vi "Control - PID Control.vi"() -> ()   [LabVIEW 2013, in "PID Control Workspace Object.lvlib"]
doc: "Sample numeric display item."
uses:
  Control Workspace Object Support.llb/PID Control Workspace Object.lvlib
  NationalInstruments.VeriStand.SystemStorage
  NationalInstruments.VeriStand.ClientAPI
  Control Workspace Object Support.llb/Constants.vi
  Control Workspace Object Support.llb/Control Addon Shared.lvlib
  Control Workspace Object Support.llb/NI_VS Workspace ExecutionAPI.lvlib
panel:
  in  "Manual Output":dbl
  in  "Manual Control":bool
  in  "Setpoint":dbl
  in  "NIVS.System Definition Root":refnum<k24>
  in  "NIVS.Gateway IP Address":string
  in  "Hold":bool
  in  "Autoscale Y":bool=TRUE
  in  "Autoscale X":bool=TRUE
  out "Chart":waveform(dbl)[](graph)
  out "Control Name":string
  in  "Item.Data":T1
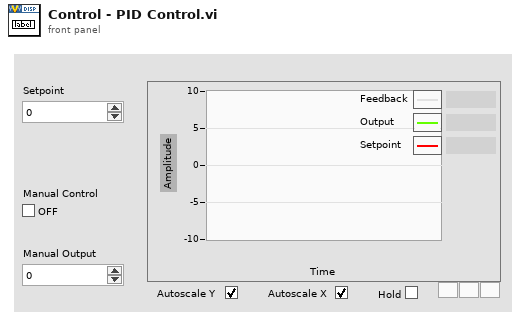
[diagram p1: front panel]
types:
  T1 = cluster{"Template VI":string, "Position X":i32, "Position Y":i32, "Custom":string, "Show Title Bar":bool, "ID":i32, "Always On Top":bool, "Allow Resize":bool, "Allow Minimize":bool, "Allow Close":bool, "Size to Screen":bool, "Screen.ID":i32, "State":enum16{"Normal", "New"}, "Title":string, "Window Bounds":cluster{"[0]":i16, "[1]":i16, "[2]":i16, "[3]":i16}, "Channel Ref":u64, "Unit":string, "Default Units?":bool, "Flash Limit?":bool, "Color 1":u32, "Color 2":u32, "Color 3":u32, "Color 4":u32, "Bck Color":u32, "Fore Color":u32, "Limit 1":dbl, "Limit 2":dbl, "Limit 3":dbl, "Limit 4":dbl, "Limit Mode 1":i32, "Limit Mode 2":i32, "Limit Mode 3":i32, "Limit Mode 4":i32, "Scale Precision":i32, "Scale Min":dbl, "Scale Max":dbl, "Format":i32, "Precision":i32, "Background Type":i32, "IDs":i32[], "Units":string[], "Labels":string[], "Scale Factor":dbl, "Scale Offset":dbl, "YScale Index":u32[], "XScale":cluster{"Format":u8, "Precision":u8, "Fit":u8, "Label":string, "Use Default Label":bool, "Label Visible":bool, "Min":dbl, "Max":dbl}, "YScales":cluster{"Format":u8, "Precision":u8, "Fit":u8, "Label":string, "Use Default Label":bool, "Label Visible":bool, "Min":dbl, "Max":dbl}[], "Plots":cluster{"Bar Style":u8, "Fill To":i16, "Fill/PtColor":u32, "Line Style":u8, "Line Width":u8, "Color":u32, "Interp":u8, "Point Style":u8}[], "Update Period":dbl, "History Length":dbl, "My.Ref":refnum<vi>, "Is Control?":bool, "Channel Paths":string[], "Custom Data":variant}
  T2 = enum8{"Idle", "Start Acq", "Run", "Stop Acq", "Exit"}
  T3 = cluster{"Action":enum8{"Idle", "Start Acq", "Run", "Stop Acq", "Exit"}, "Channels":string[]}
  T4 = cluster{"Initialized Waveform":waveform(dbl)[], "VS UDP Session":refnum<k24>, "Channel IDs":i32[], "Packet IDs":i32[], "Max Packet Size":i32, "UDP Ref":refnum<k16>}
  T5 = cluster{"Cached":cluster{"Path":string}, "Found?":bool, "UDP Channels":string[], "Connected?":bool, "Previous Values":dbl[], "Slow Channels":string[]}
  T6 = cluster{"Operation":enum16{"SetCustomData", "DeleteItem"}, "Data":variant}
  T7 = cluster{"CustDatRef":refnum<user-event>, "EvtRef":refnum<k27>}
  T8 = cluster{"Event Registration Refnum":refnum<event-registration>, "SystemChangeEventRef":refnum<event-registration>}
  T9 = cluster{"ID":i32, "t0":dbl, "dt":dbl, "Channel IDs":i32[], "Channel Data":dbl[][], "Sample Offset":u64}
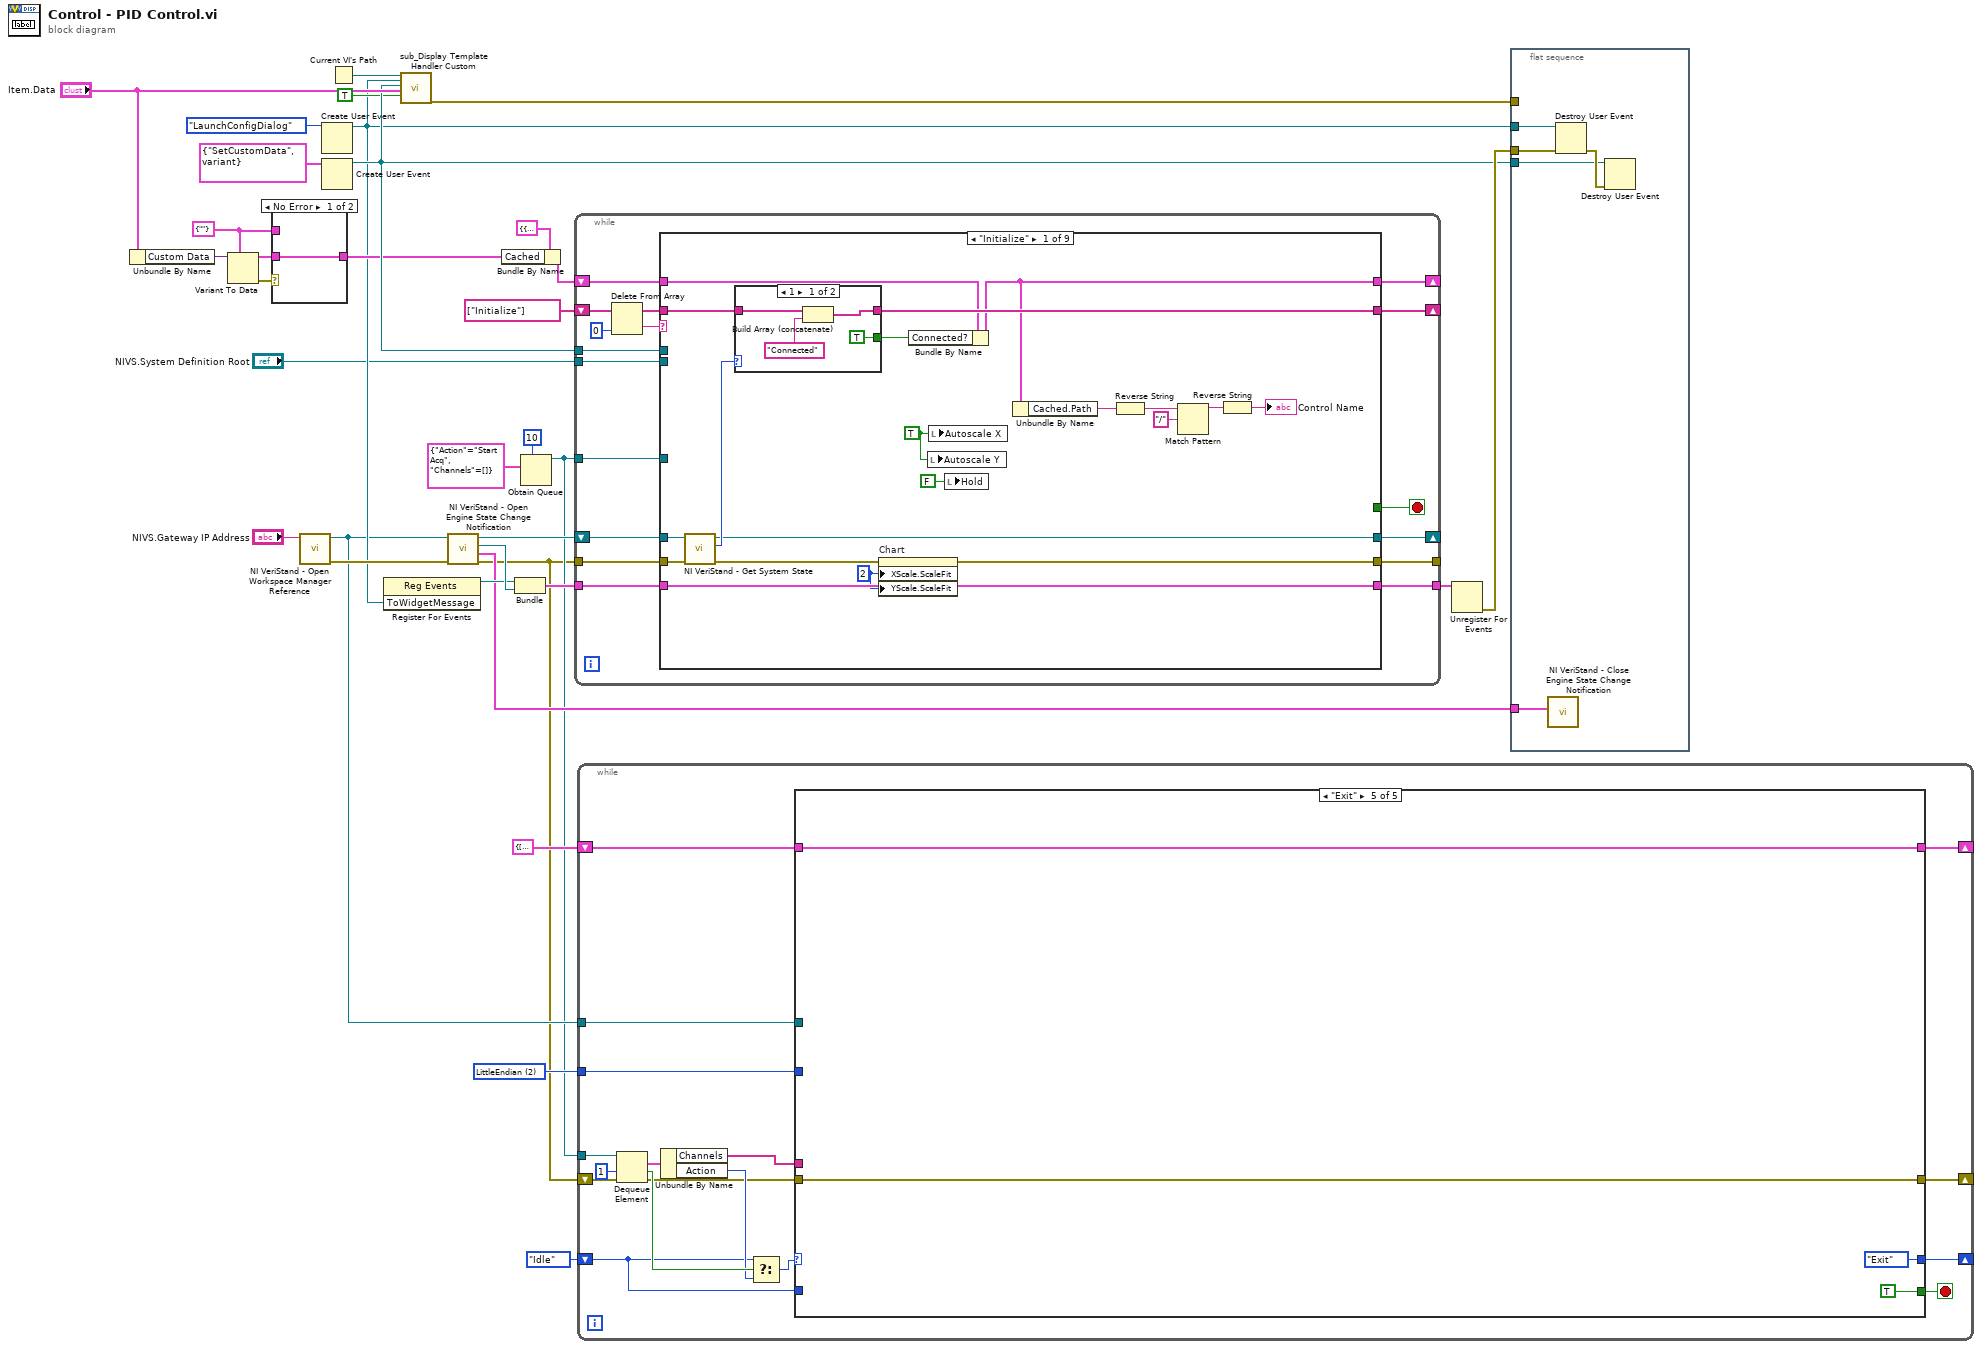
[diagram p0: block diagram]
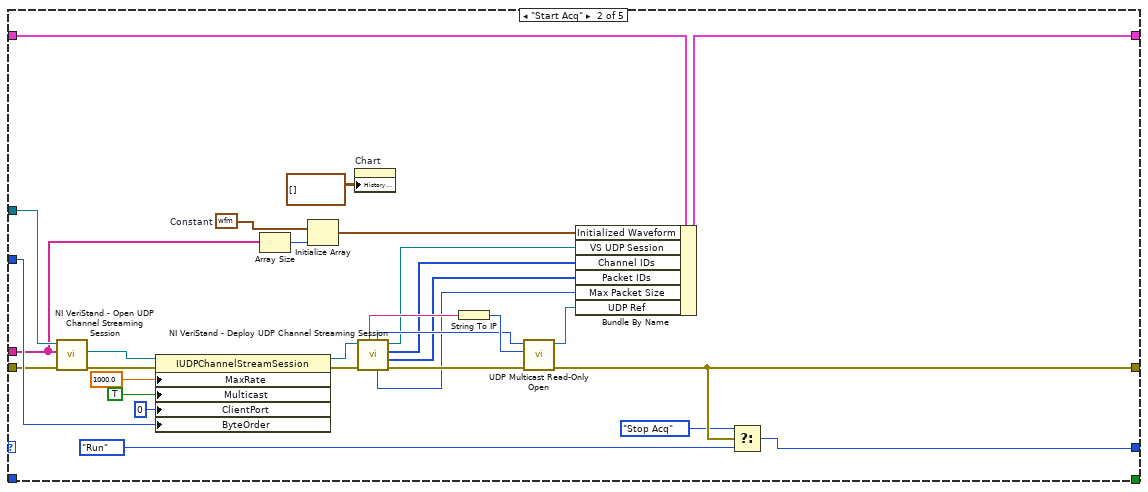
[diagram p3: hidden frame]
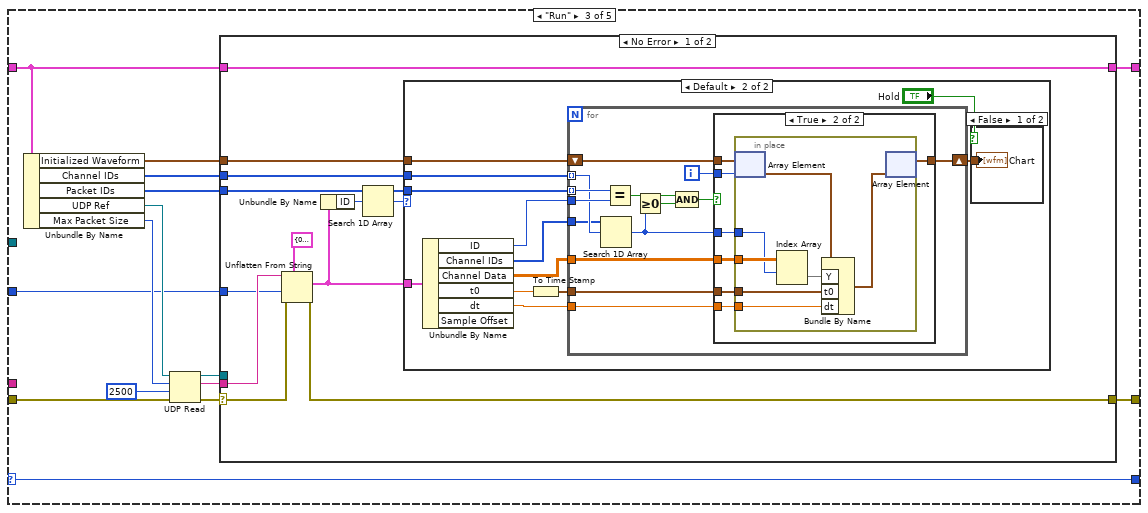
[diagram p4: hidden frame]
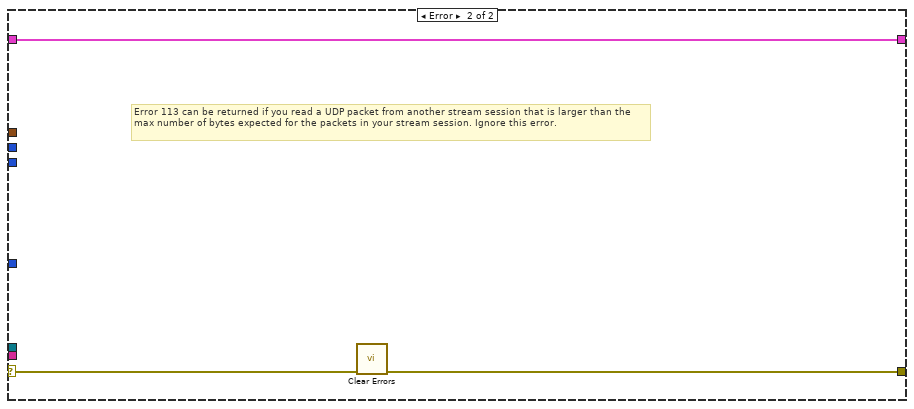
[diagram p8: hidden frame]
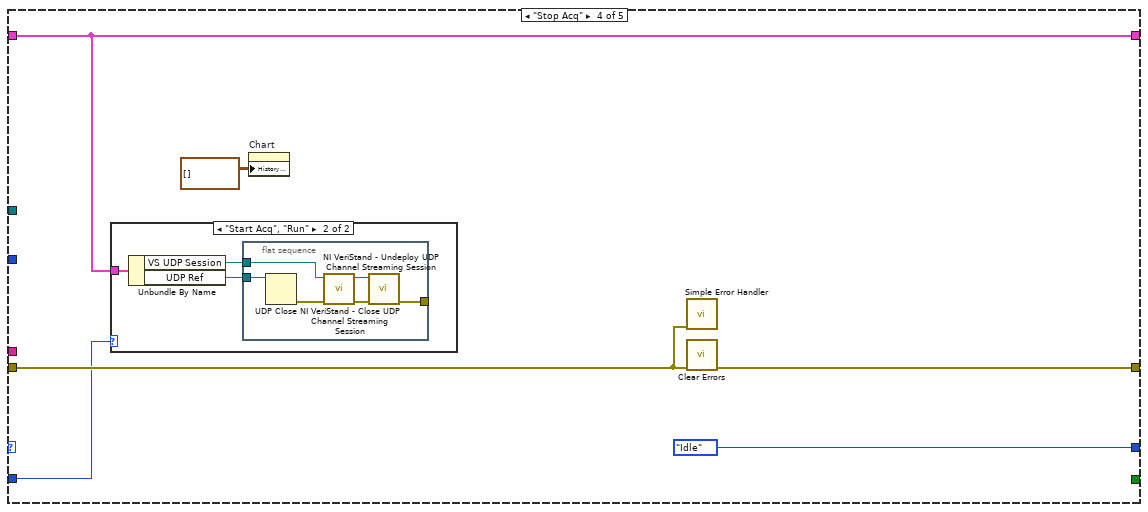
[diagram p9: hidden frame]
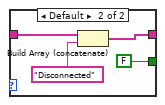
[diagram p12: hidden frame]
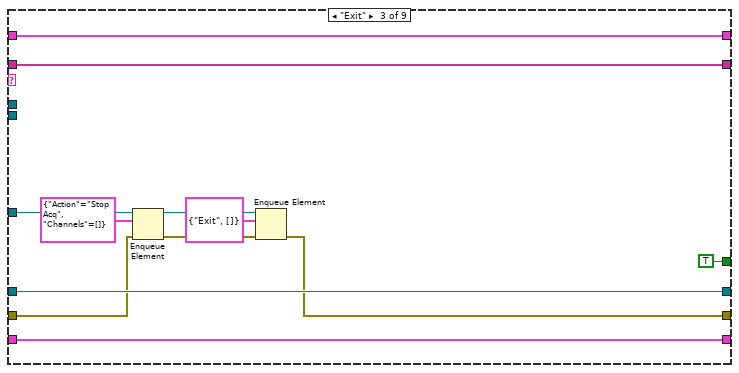
[diagram p14: hidden frame]
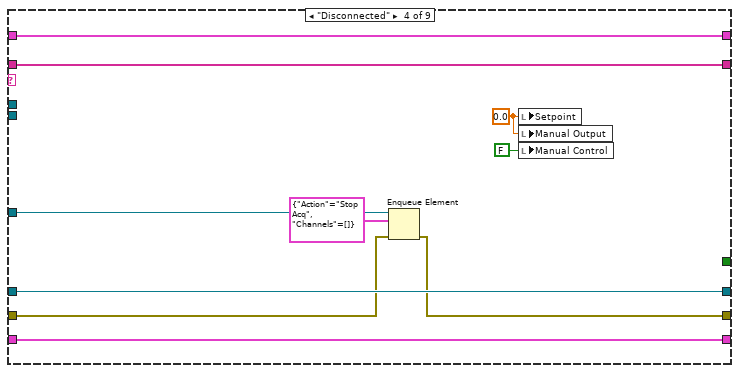
[diagram p15: hidden frame]
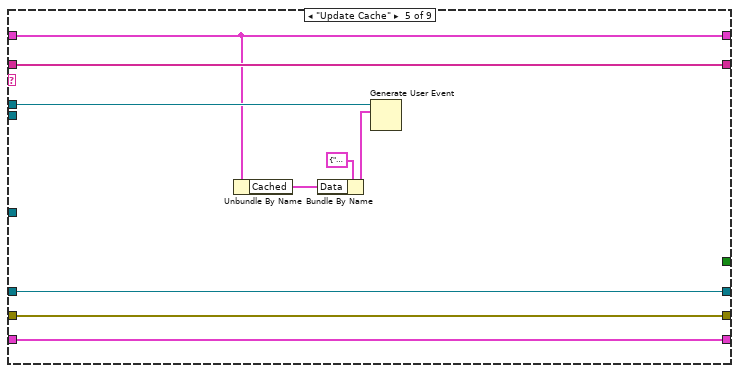
[diagram p16: hidden frame]
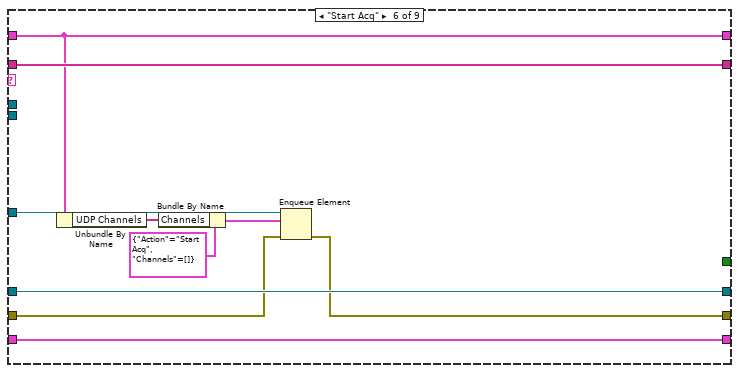
[diagram p17: hidden frame]
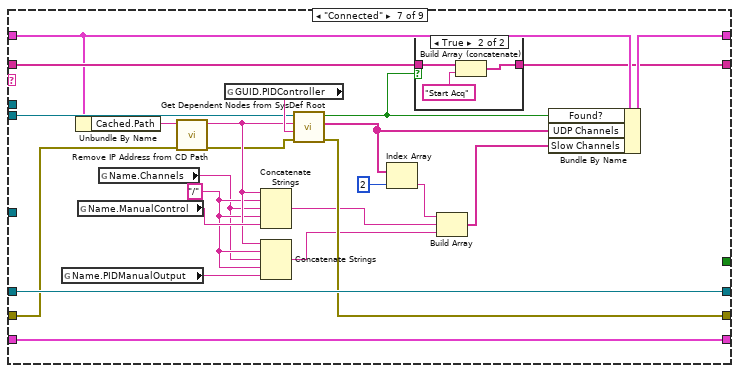
[diagram p18: hidden frame]
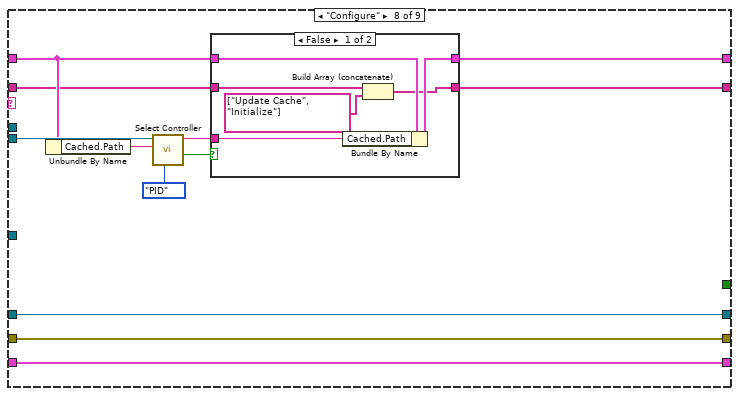
[diagram p20: hidden frame]
diagram:
  w6 = 2 items=["BigEndian", "NativeHostOrder", "LittleEndian"] ("Byte Order")
  w14 = cluster{"Path":string} {"Path"=""}
  n1 = Unbundle By Name("Item.Data") -> ("Custom Data"=w18:variant)
  n2 = Variant To Data(type=w14, Variant=w18) -> (data=w15:cluster{"Path":string}, error out=w16:errorcluster)  [unwired: 1 in]
  n3 = case shown="No Error" w16 {
    tunnel: w15 -> [w35 _]
    tunnel: [w35 w36] -> w11
    tunnel: w14 -> [_ w36]
    frame No Error {
    }
    frame Error {
    }
  }
  n4 = call "NI VeriStand - Open Workspace Manager Reference.vi"("Gateway IP Address (\"\": localhost)"="NIVS.Gateway IP Address") -> ("error out"=w25:errorcluster, "WorkspaceManager"=w8:refnum<k24>)  [unwired: 9 in]
  n5 = Create User Event(user event datatype=enum16{"Stop", "LaunchConfigDialog"}."LaunchConfigDialog" ("ToWidgetMessage")) -> (user event=w10:refnum<user-event>)  [unwired: 1 in, 1 out]
  n6 = Create User Event(user event datatype=T6 {"Operation"=enum."SetCustomData", "Data"=variant} ("Data")) -> (user event=w28:refnum<user-event>)  [unwired: 1 in, 1 out]
  n7 = Current VI's Path() -> (path=w30:path)
  n8 = register-events(w10) -> (reference out=w23:refnum<event-registration>)  [unwired: 2 in, 1 out]
  n9 = call "sub_Display Template Handler Custom.vi"("Parent.Path"=w30, "ToWidgetEvent"=w10, "ToWorkspace"=w28, "Item.Data"="Item.Data", "Resizable"=TRUE) -> ("error out"=w34:errorcluster)  [unwired: 14 in]
  n10 = call "NI VeriStand - Open Engine State Change Notification.vi"("error in (no error)"=w25, "WorkspaceManager in"=w8) -> ("error out"=w1:errorcluster, "SystemStateRefs"=w21:T7, "SystemChangeEventRef"=w24:refnum<event-registration>, "WorkspaceManager out"=w19:refnum<k24>)  [unwired: 6 in]
  n11 = Bundle By Name(cluster=T5 {"Cached"={"Path"=""}, "Found?"=FALSE, "UDP Channels"=[], "Connected?"=FALSE, "Previous Values"=[0.0, 0.0, 0.0], "Slow Channels"=[]}, "Cached"=w11) -> (w12:T5)
  n12 = Bundle("Event Registration Refnum"=w23, "SystemChangeEventRef"=w24) -> (w22:T8)  [unwired: 1 in]
  n13 = Obtain Queue(max queue size (-1, unlimited)=10, element data type=T3 {"Action"=enum."Start Acq", "Channels"=[]}) -> (queue out=w3:refnum<queue>)  [unwired: 3 in, 2 out]
  n14 = while {
    tunnel: w22 -> [w53]
    tunnel: w28 -> [w51]
    shift-right: [w45] -> _
    shift-left: string[] ["Initialize"] -> [w49]
    shift-right: [w43] -> _
    shift-left: w19 -> [w42]
    tunnel: w1 -> [w47]
    tunnel: [w44] -> w17
    tunnel: [w40] -> _
    shift-right: [w39] -> _
    shift-left: w12 -> [w41]
    tunnel: "NIVS.System Definition Root" -> [w38]
    tunnel: w3 -> [w37]
    stop <- w52 stop-if-true
    n15 = Delete From Array(array=w49, index=0) -> (deleted portion=w48:string, array with subset deleted=w46:string[])  [unwired: 1 in]
    n16 = case shown="\"Initialize\"" w48 {
      tunnel: w53 -> [w67 w85 w97 w107 w116 w126 w150 w167 w186]
      tunnel: [_ _ TRUE _ _ _ _ _ _] -> w52
      tunnel: [w69 w86 w98 w108 w117 w127 w133 w157 w183] -> w45
      tunnel: w51 -> [_ _ _ _ w113 _ _ _ _]
      tunnel: w47 -> [w72 w83 w89 w103 w114 w119 w137 w165 w179]
      tunnel: w46 -> [w70 w86 w98 w108 w117 w127 w151 w156 w182]
      tunnel: [w67 w85 w97 w107 w116 w126 w150 w167 w184] -> w44
      tunnel: [w68 w84 w96 w106 w115 w125 w149 w166 w180] -> w43
      tunnel: w42 -> [w71 w84 w96 w106 w115 w125 w149 w166 w181]
      tunnel: w41 -> [w61 w82 w95 w105 w110 w124 w145 w161 w176]
      tunnel: [w55 w83 w88 w102 w114 w118 w148 w165 w178] -> w40
      tunnel: [w60 w82 w95 w105 w110 w124 w144 w160 w177] -> w39
      tunnel: w38 -> [_ _ _ _ _ _ w146 w163 _]
      tunnel: w37 -> [_ _ w94 w104 _ w123 _ _ _]
      frame "Initialize" {
        w57 = u8 2 ("X Scale.Scale Fit")
        w58 = TRUE ("Autoscale X")
        n17 = call "NI VeriStand - Get System State.vi"("error in (no error)"=w72, "WorkspaceManager in"=w71) -> ("error out"=w56:errorcluster, "System State"=w73:u8, "WorkspaceManager  out"=w68:refnum<k24>)  [unwired: 5 in, 2 out]
        n18 = case shown="1" w73 {
          tunnel: w70 -> [w77 w81]
          tunnel: [w76 w80] -> w69
          tunnel: [TRUE FALSE] -> w59
          frame 1 {
            n19 = Build Array (concatenate)(w77, "Connected") -> (w76:string[])
          }
          frame Default {
            n20 = Build Array (concatenate)(w81, "Disconnected") -> (w80:string[])
          }
        }
        n21 = property on="Chart" class="WFChart (strict)"(error in=w56, "XScale.ScaleFit"=w57, "YScale.ScaleFit"=w57) -> (error out=w55:errorcluster)  [unwired: 1 in, 1 out]
        n22 = Bundle By Name(cluster=w61, "Connected?"=w59) -> (w60:T5)
        n23 = local write "Autoscale Y"(w58) -> ()
        n24 = local write "Autoscale X"(w58) -> ()
        n25 = local write "Hold"(FALSE ("Hold")) -> ()
        n26 = Unbundle By Name(w60) -> ("Cached.Path"=w63:string)
        n27 = Reverse String(1:w63) -> (0:w66:string)
        n28 = Match Pattern(string=w66, regular expression="/") -> (before substring=w62:string)  [unwired: 1 in, 3 out]
        n29 = Reverse String(1:w62) -> (0:→"Control Name":string)
      }
      frame Default {
      }
      frame "Exit" {
        n30 = Enqueue Element(queue=w94, element=T3 {"Action"=enum."Stop Acq", "Channels"=[]}, error in (no error)=w89) -> (queue out=w92:refnum<queue>, error out=w90:errorcluster)  [unwired: 1 in, 1 out]
        n31 = Enqueue Element(queue=w92, element=T3 {"Action"=enum."Exit", "Channels"=[]}, error in (no error)=w90) -> (error out=w88:errorcluster)  [unwired: 1 in, 2 out]
      }
      frame "Disconnected" {
        w100 = 0.0 ("Setpoint")
        n32 = Enqueue Element(queue=w104, element=T3 {"Action"=enum."Stop Acq", "Channels"=[]}, error in (no error)=w103) -> (error out=w102:errorcluster)  [unwired: 1 in, 2 out]
        n33 = local write "Setpoint"(w100) -> ()
        n34 = local write "Manual Output"(w100) -> ()
        n35 = local write "Manual Control"(FALSE ("Manual Control")) -> ()
      }
      frame "Update Cache" {
        n36 = Unbundle By Name(w110) -> ("Cached"=w109:cluster{"Path":string})
        n37 = Bundle By Name(cluster=T6 {"Operation"=enum."SetCustomData", "Data"=variant} ("event data"), "Data"=w109) -> (w111:T6)
        n38 = Generate User Event(user event=w113, event data cluster=w111) -> ()  [unwired: 2 in, 2 out]
      }
      frame "Start Acq" {
        n39 = Unbundle By Name(w124) -> ("UDP Channels"=w121:string[])
        n40 = Bundle By Name(cluster=T3 {"Action"=enum."Start Acq", "Channels"=[]}, "Channels"=w121) -> (w120:T3)
        n41 = Enqueue Element(queue=w123, element=w120, error in (no error)=w119) -> (error out=w118:errorcluster)  [unwired: 1 in, 2 out]
      }
      frame "Connected" {
        w130 = "/" ("string")
        n42 = global read "Constants.vi" "Name.PIDManualOutput"() -> (w140:string)
        n43 = Unbundle By Name(w145) -> ("Cached.Path"=w143:string)
        n44 = global read "Constants.vi" "Name.ManualControl"() -> (w142:string)
        n45 = global read "Constants.vi" "Name.Channels"() -> (w129:string)
        n46 = call "Remove IP Address from CD Path.vi"("error in (no error)"=w137, "CD Path"=w143) -> ("error out"=w136:errorcluster, "Path"=w141:string)  [unwired: 8 in]
        n47 = global read "Constants.vi" "GUID.PIDController"() -> (w147:string)
        n48 = Concatenate Strings(w141, w130, w129, w130, w142) -> (w139:string)
        n49 = Concatenate Strings(w141, w130, w129, w130, w140) -> (w138:string)
        n50 = call "Get Dependent Nodes from SysDef Root.vi"("error in (no error)"=w136, "GUID"=w147, "Path"=w141, "SysDef Ref"=w146) -> ("error out"=w148:errorcluster, "Channels"=w132:string[], "Found"=w128:bool)  [unwired: 5 in]
        n51 = Index Array(array=w132, index=2) -> (element=w134:string)
        n52 = case shown="True" w128 {
          tunnel: w151 -> [w152 w155]
          tunnel: [w152 w154] -> w133
          frame False {
          }
          frame True {
            n53 = Build Array (concatenate)(w155, "Start Acq") -> (w154:string[])
          }
        }
        n54 = Build Array(w134, w139, w138) -> (w131:string[])
        n55 = Bundle By Name(cluster=w145, "Found?"=w128, "UDP Channels"=w132, "Slow Channels"=w131) -> (w144:T5)
      }
      frame "Configure" {
        n56 = Unbundle By Name(w161) -> ("Cached.Path"=w162:string)
        n57 = call "Select Controller.vi"("Type"=enum16{"PID", "Industrial"}."PID", "CD Path"=w162, "NIVS.System Definition Root"=w163) -> ("Cancelled?"=w159:bool, "Custom Device Path Out"=w158:string)  [unwired: 6 in, 1 out]
        n58 = case shown="False" w159 {
          tunnel: w161 -> [w173 w174]
          tunnel: [w172 w174] -> w160
          tunnel: w158 -> [w171 _]
          tunnel: [w169 w175] -> w157
          tunnel: w156 -> [w170 w175]
          frame False {
            n59 = Bundle By Name(cluster=w173, "Cached.Path"=w171) -> (w172:T5)
            n60 = Build Array (concatenate)(w170, string[] ["Update Cache", "Initialize"]) -> (w169:string[])
          }
          frame True {
          }
        }
      }
      frame "" {
        n61 = event shown="[1] \"Autoscale Y\", \"Autoscale X\": Value Change" {
          selector: w186 -> [_ _ _ _ _]
          dyn-events: [_ _ _ _ _] -> w184
          timeout: 100 -> [_ _ _ _ _]
          tunnel: [w203 w225 w242 w271 w291] -> w183
          tunnel: w182 -> [w203 w225 w242 w272 w290]
          tunnel: w181 -> [w200 w224 w235 w275 w292]
          tunnel: [w199 w224 w234 w274 w292] -> w180
          tunnel: w179 -> [w202 w218 w237 w277 w289]
          tunnel: [w201 w217 w236 w276 w289] -> w178
          tunnel: [w196 w223 w230 w269 w288] -> w177
          tunnel: w176 -> [w197 w223 w230 w270 w288]
          event Timeout {
            n62 = event-data() -> ()  [unwired: 2 out]
            n63 = Unbundle By Name(w197) -> ("Found?"=w189:bool, "Connected?"=w195:bool, "Slow Channels"=w198:string[])
            n64 = Compound Arithmetic op=AND(w189, w195) -> (w190:bool)
            n65 = case shown="True" w190 {
              tunnel: w202 -> [w206 w212]
              tunnel: [w206 w211] -> w201
              tunnel: w200 -> [w205 w210]
              tunnel: [w205 w209] -> w199
              tunnel: w198 -> [_ w208]
              tunnel: [dbl[] [0.0, 0.0, 0.0] ("Values") w207] -> w194
              frame False {
              }
              frame True {
                n66 = call "NI VeriStand - Get Multiple Channel Values.vi"("error in (no error)"=w212, "Channels"=w208, "WorkspaceManager in"=w210) -> ("error out"=w211:errorcluster, "Values"=w207:dbl[], "WorkspaceManager out"=w209:refnum<k24>)  [unwired: 6 in]
              }
            }
            n67 = Index Array(array=w194) -> (element #1=w193:dbl, element #2=w188:dbl, element #3=w187:dbl)  [unwired: 3 in]
            n68 = To Long Integer(number=w188) -> (32bit integer=w192:i32)
            n69 = Not Equal To 0?(x=w192) -> (x != 0?=w191:bool)
            n70 = local write "Setpoint"(w193) -> ()
            n71 = local write "Manual Control"(w191) -> ()
            n72 = local write "Manual Output"(w187) -> ()
            n73 = Bundle By Name(cluster=w197, "Previous Values"=w194) -> (w196:T5)
          }
          event "Autoscale Y", "Autoscale X": Value Change {
            n74 = event-data() -> ()  [unwired: 2 out]
            n75 = Select(t=u8 2, s="Autoscale X", f=u8 0 ("X Scale.Scale Fit")) -> (s? t:f=w220:u8)
            n76 = Select(t=u8 2, s="Autoscale Y", f=u8 0 ("X Scale.Scale Fit")) -> (s? t:f=w213:u8)
            n77 = property on="Chart" class="WFChart (strict)"(error in=w218, "XScale.ScaleFit"=w220, "YScale.ScaleFit"=w213) -> (error out=w217:errorcluster)  [unwired: 1 in, 1 out]
          }
          event "Setpoint", "Manual Control", "Manual Output": Value Change {
            n78 = event-data() -> ()  [unwired: 2 out]
            n79 = Unbundle By Name(w230) -> ("Found?"=w228:bool, "Connected?"=w232:bool, "Previous Values"=w231:dbl[], "Slow Channels"=w233:string[])
            n80 = Boolean To (0,1)(Boolean="Manual Control") -> (0, 1=w227:i16)
            n81 = Build Array("Setpoint", w227, "Manual Output") -> (w238:dbl[])
            n82 = Not Equal?(x=w231, y=w238) -> (x != y?=w241:bool[])
            n83 = Compound Arithmetic op=AND(w228, w232) -> (w229:bool)
            n84 = case shown="True" w229 {
              tunnel: w241 -> [_ w251]
              tunnel: w238 -> [_ w250]
              tunnel: w237 -> [w244 w249]
              tunnel: [w244 w248] -> w236
              tunnel: w235 -> [w243 w247]
              tunnel: [w243 w246] -> w234
              tunnel: w233 -> [_ w245]
              frame False {
              }
              frame True {
                n85 = for {
                  shift-right: [w257] -> w248
                  shift-left: w249 -> [w258]
                  shift-right: [w256] -> w246
                  shift-left: w247 -> [w255]
                  tunnel: w251 -> [w254] mode=indexing
                  tunnel: w250 -> [w253] mode=indexing
                  tunnel: w245 -> [w252] mode=indexing
                  n86 = case shown="False" w254 {
                    tunnel: w258 -> [w260 w266]
                    tunnel: [w260 w265] -> w257
                    tunnel: [w259 w264] -> w256
                    tunnel: w255 -> [w259 w263]
                    tunnel: w253 -> [_ w262]
                    tunnel: w252 -> [_ w261]
                    frame False {
                    }
                    frame True {
                      n87 = call "NI VeriStand - Set Single Channel Value.vi"("error in (no error)"=w266, "Value"=w262, "Channel"=w261, "WorkspaceManager in"=w263) -> ("error out"=w265:errorcluster, "WorkspaceManager out"=w264:refnum<k24>)  [unwired: 6 in]
                    }
                  }
                }
              }
            }
          }
          event User Event {
            n88 = event-data() -> ()  [unwired: 2 out]
            n89 = call "NI VeriStand - Get System State.vi"("error in (no error)"=w277, "WorkspaceManager in"=w275) -> ("error out"=w276:errorcluster, "System State"=w273:u8, "WorkspaceManager  out"=w274:refnum<k24>)  [unwired: 5 in, 2 out]
            n90 = case shown="Default" w273 {
              tunnel: w272 -> [w282 w287]
              tunnel: [w281 w286] -> w271
              tunnel: [w279 w284] -> w268
              tunnel: w270 -> [w279 w284]
              tunnel: [TRUE FALSE] -> w267
              frame 1 {
                n91 = Build Array (concatenate)(w282, "Connected") -> (w281:string[])
              }
              frame Default {
                n92 = Build Array (concatenate)(w287, "Disconnected") -> (w286:string[])
              }
            }
            n93 = Bundle By Name(cluster=w268, "Connected?"=w267) -> (w269:T5)
          }
          event User Event {
            n94 = event-data() -> ("ToWidgetMessage"=w293:enum16{"Stop", "LaunchConfigDialog"})  [unwired: 1 out]
            n95 = case shown="\"Stop\"" w293 {
              tunnel: [w294 w296 w299] -> w291
              tunnel: w290 -> [w294 w297 w300]
              frame Default {
              }
              frame "Stop" {
                n96 = Build Array (concatenate)(w297, "Exit") -> (w296:string[])
              }
              frame "LaunchConfigDialog" {
                n97 = Build Array (concatenate)(w300, "Configure") -> (w299:string[])
              }
            }
          }
        }
      }
    }
  }
  n98 = while {
    tunnel: w8 -> [w317]
    tunnel: w6 -> [w315]
    tunnel: w3 -> [w314]
    shift-right: [w308] -> _
    shift-left: T2."Idle" ("Action") -> [w301]
    shift-right: [w307] -> _
    shift-left: T4 {"Initialized Waveform"=[], "VS UDP Session"=refnum, "Channel IDs"=[], "Packet IDs"=[], "Max Packet Size"=0, "UDP Ref"=refnum} -> [w316]
    shift-right: [w304] -> _
    shift-left: w1 -> [w303]
    stop <- w306 stop-if-true
    n99 = Dequeue Element(queue=w314, timeout in ms (-1)=1, error in (no error)=w303) -> (element=w313:T3, timed out?=w311:bool, error out=w305:errorcluster)  [unwired: 1 out]
    n100 = Unbundle By Name(w313) -> ("Channels"=w302:string[], "Action"=w310:T2)
    n101 = Select(t=w301, s=w311, f=w310) -> (s? t:f=w309:T2)
    n102 = case shown="\"Exit\"" w309 {
      selector: w309 -> [w318 _ w354 _ _]
      tunnel: w317 -> [_ w338 _ _ _]
      tunnel: w316 -> [w320 w337 w355 w428 w439]
      tunnel: w315 -> [_ w330 w351 _ _]
      tunnel: [w320 w329 w356 w428 w439] -> w307
      tunnel: [w318 w324 w354 T2."Idle" ("Action") T2."Exit" ("Action")] -> w308
      tunnel: [_ _ _ _ TRUE] -> w306
      tunnel: w305 -> [w319 w328 w353 w426 w438]
      tunnel: [w319 w327 w352 w425 w438] -> w304
      tunnel: w302 -> [_ w322 _ _ _]
      tunnel: w301 -> [_ _ _ w424 _]
      frame "Idle" {
      }
      frame "Start Acq" {
        w344 = waveform(dbl) {"t0"=timestamp(0 s since 1904-01-01), "dt"=1.0, "Y"=[]}  # Constant
        n103 = call "NI VeriStand - Open UDP Channel Streaming Session.vi"("error in (no error)"=w328, "Channels"=w322, "WorkspaceManager in"=w338) -> ("error out"=w348:errorcluster, "UDPChannelStreamSession out"=w345:refnum<k24>)  [unwired: 6 in, 1 out]
        n104 = property class="IUDPChannelStreamSession"(reference=w345, error in=w348, "MaxRate"=1000.0, "Multicast"=TRUE, "ClientPort"=u16 0, "ByteOrder"=w330) -> (reference out=w347:refnum<k24>, error out=w346:errorcluster)
        n105 = Array Size(array=w322) -> (size(s)=w343:i32)
        n106 = Initialize Array(w344, w343) -> (w336:waveform(dbl)[])
        n107 = property on="Chart" class="WFChart (strict)"("History Data"=waveform(dbl)[][] []) -> ()  [unwired: 2 in, 2 out]
        n108 = call "NI VeriStand - Deploy UDP Channel Streaming Session.vi"("error in (no error)"=w346, "UDPChannelStreamSession in"=w347) -> ("error out"=w340:errorcluster, "Packet IDs"=w333:i32[], "Channel IDs"=w334:i32[], "UDPChannelStreamSession out"=w335:refnum<k24>, "Max Packet Size"=w332:i32, "Port"=w341:u16, "UDP Multicast Address"=w339:string)  [unwired: 3 in]
        n109 = String To IP(1:w339) -> (0:w342:u32)
        n110 = call "UDP Multicast Read-Only Open.vi"("error in (no error)"=w340, "multicast addr"=w342, "port"=w341) -> ("error out"=w327:errorcluster, "connection ID"=w331:refnum<k16>)  [unwired: 6 in, 1 out]
        n111 = Bundle By Name(cluster=w337, "Initialized Waveform"=w336, "VS UDP Session"=w335, "Channel IDs"=w334, "Packet IDs"=w333, "Max Packet Size"=w332, "UDP Ref"=w331) -> (w329:T4)
        n112 = Select(t=T2."Stop Acq", s=w327, f=T2."Run" ("Action")) -> (s? t:f=w324:T2)
      }
      frame "Run" {
        n113 = Unbundle By Name(w355) -> ("Initialized Waveform"=w361:waveform(dbl)[], "Channel IDs"=w360:i32[], "Packet IDs"=w359:i32[], "UDP Ref"=w358:refnum<k16>, "Max Packet Size"=w357:i32)
        n114 = UDP Read(connection ID=w358, max size (548)=w357, timeout ms (25000)=2500, 8:w353) -> (data out=w363:string, error out=w364:errorcluster, 3:w365:refnum<k16>)  [unwired: 2 out]
        n115 = case shown="No Error" w364 {
          selector: w364 -> [w376 w422]
          tunnel: w359 -> [w371 _]
          tunnel: w363 -> [w374 _]
          tunnel: w360 -> [w373 _]
          tunnel: w361 -> [w372 _]
          tunnel: [w377 w420] -> w352
          tunnel: w365 -> [_ _]
          tunnel: w351 -> [w367 _]
          tunnel: [w366 w421] -> w356
          tunnel: w355 -> [w366 w421]
          frame No Error {
            n116 = Unflatten From String(type=T9 {"ID"=0, "t0"=0.0, "dt"=0.0, "Channel IDs"=[], "Channel Data"=[], "Sample Offset"=0} ("UDP Data Packet"), binary string=w374, byte order (0:big-endian, network order)=w367, error in (no error)=w376) -> (value=w368:T9, error out=w377:errorcluster)  [unwired: 1 in, 1 out]
            n117 = Unbundle By Name(w368) -> ("ID"=w369:i32)
            n118 = Search 1D Array(1D array=w371, element=w369) -> (index of element=w370:i32)  [unwired: 1 in]
            n119 = case shown="Default" w370 {
              tunnel: w373 -> [_ w389]
              tunnel: w372 -> [_ w388]
              tunnel: w371 -> [_ w386]
              tunnel: w368 -> [_ w385]
              frame -1 {
                # "This is a packet from a different UDP session. Ignore it."
              }
              frame Default {
                n120 = Unbundle By Name(w385) -> ("ID"=w384:i32, "Channel IDs"=w383:i32[], "Channel Data"=w382:dbl[][], "t0"=w381:dbl, "dt"=w380:dbl)  [unwired: 1 out]
                n121 = To Time Stamp(1:w381) -> (0:w387:timestamp)
                n122 = for {
                  tunnel: w389 -> [w402] mode=indexing
                  tunnel: w386 -> [w404] mode=indexing
                  tunnel: w384 -> [w403]
                  tunnel: w382 -> [w396]
                  tunnel: w383 -> [w395]
                  shift-right: [w391] -> w379
                  shift-left: w388 -> [w394]
                  tunnel: w387 -> [w393]
                  tunnel: w380 -> [w392]
                  i -> [w397]
                  n123 = Search 1D Array(1D array=w395, element=w402) -> (index of element=w398:i32)  [unwired: 1 in]
                  n124 = Equal?(x=w404, y=w403) -> (x = y?=w401:bool)
                  n125 = Greater Or Equal To 0?(x=w398) -> (x >= 0?=w400:bool)
                  n126 = Compound Arithmetic op=AND(w401, w400) -> (w399:bool)
                  n127 = case shown="True" w399 {
                    tunnel: w398 -> [_ w410]
                    tunnel: w397 -> [_ w406]
                    tunnel: w396 -> [_ w411]
                    tunnel: w394 -> [w405 w412]
                    tunnel: w393 -> [_ w409]
                    tunnel: w392 -> [_ w408]
                    tunnel: [w405 w407] -> w391
                    frame False {
                      # "This channel is not in this UDP Data Packet."
                    }
                    frame True {
                      n128 = in-place {
                        in-place-border: w411 -> [w418]
                        in-place-border: w410 -> [w417]
                        in-place-border: w409 -> [w415]
                        in-place-border: w408 -> [w414]
                        n129 = in-place-array #1(w412, w406) -> (w419:waveform(dbl))
                        n130 = Index Array(array=w418, index (row)=w417) -> (element=w416:dbl[])  [unwired: 1 in]
                        n131 = Bundle By Name(cluster=w419, "Y"=w416, "t0"=w415, "dt"=w414) -> (w413:waveform(dbl))
                        n132 = in-place-array #1(w413) -> (w407:waveform(dbl)[])  [unwired: 1 out]
                      }
                    }
                  }
                }
                n133 = case shown="False" "Hold" {
                  tunnel: w379 -> [w390 _]
                  frame False {
                    "Chart" <- w390
                  }
                  frame True {
                  }
                }
              }
            }
          }
          frame Error {
            # "Error 113 can be returned if you read a UDP packet from another stream session that is larger than the max number of bytes expected for the packets in your stream session. Ignore this error."
            n134 = call "Clear Errors.vi"("error in (no error)"=w422) -> ("error out"=w420:errorcluster)  [unwired: 6 in]
          }
        }
      }
      frame "Stop Acq" {
        n135 = case shown="\"Start Acq\", \"Run\"" w424 {
          tunnel: w428 -> [_ w429]
          frame Default {
          }
          frame "Start Acq", "Run" {
            n136 = Unbundle By Name(w429) -> ("VS UDP Session"=w430:refnum<k24>, "UDP Ref"=w431:refnum<k16>)
            n137 = flat-sequence {
              tunnel: w431 -> [w434]
              tunnel: w430 -> [w433]
              tunnel: [w432] -> _
              frame #0 {
                n138 = UDP Close(connection ID=w434) -> (error out=w437:errorcluster)  [unwired: 1 in, 1 out]
                n139 = call "NI VeriStand - Undeploy UDP Channel Streaming Session.vi"("error in (no error)"=w437, "UDPChannelStreamSession in"=w433) -> ("error out"=w435:errorcluster, "UDPChannelStreamSession out"=w436:refnum<k24>)  [unwired: 8 in]
                n140 = call "NI VeriStand - Close UDP Channel Streaming Session.vi"("error in (no error)"=w435, "UDPChannelStreamSession in"=w436) -> ("error out"=w432:errorcluster)  [unwired: 9 in]
              }
            }
          }
        }
        n141 = property on="Chart" class="WFChart (strict)"("History Data"=waveform(dbl)[][] []) -> ()  [unwired: 2 in, 2 out]
        n142 = call "Simple Error Handler.vi"("error in (no error)"=w426) -> ()  [unwired: 4 in, 5 out]
        n143 = call "Clear Errors.vi"("error in (no error)"=w426) -> ("error out"=w425:errorcluster)  [unwired: 6 in]
      }
      frame "Exit" {
      }
    }
  }
  n144 = Unregister For Events(event registration refnum=w17) -> (error out=w32:errorcluster)  [unwired: 1 in]
  n145 = flat-sequence {
    tunnel: w34 -> [_]
    tunnel: w32 -> [w445]
    tunnel: w10 -> [w446]
    tunnel: w28 -> [w443]
    tunnel: w21 -> [w442]
    frame #0 {
      n146 = call "NI VeriStand - Close Engine State Change Notification.vi"("SystemStateRefs"=w442) -> ()  [unwired: 10 in, 1 out]
      n147 = Destroy User Event(user event=w446, error in=w445) -> (error out=w444:errorcluster)
      n148 = Destroy User Event(user event=w443, error in=w444) -> ()  [unwired: 1 out]
    }
  }
